vi "Init Rectangle.vi"(7 "Color (RGB black)":refnum<class "Color.lvclass">=refnum, 8 "error in (no error)":errorcluster, 9 "end point":cluster{"x":i16, "y":i16}, 10 "start point":cluster{"x":i16, "y":i16}, 11 "Rectangle in":refnum<class "Rectangle.lvclass">) -> (0 "error out":errorcluster, 3 "Rectangle out":refnum<class "Rectangle.lvclass">)   [LabVIEW 2020, in "Rectangle.lvclass"]
doc: "Initialize a rectangle"
uses:
  Rectangle.lvclass
  Color/Color.lvclass
  RGB Color/RGB Color.lvclass
panel:
  # "expressionflow.com"
  # "Copyright (c) 2008 Tomi Maila. All rights reserved."
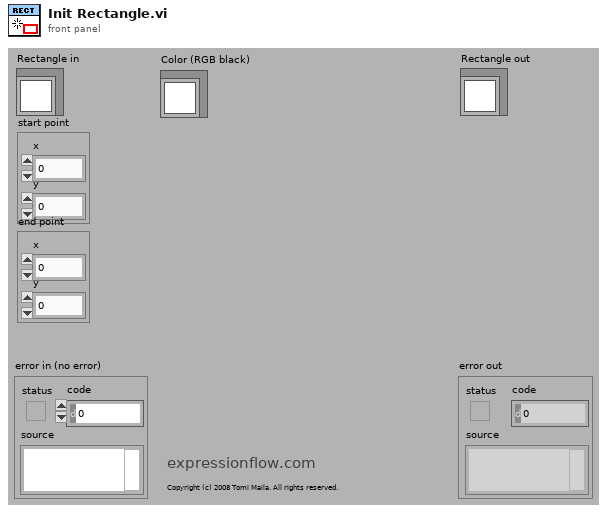
[diagram p1: front panel]
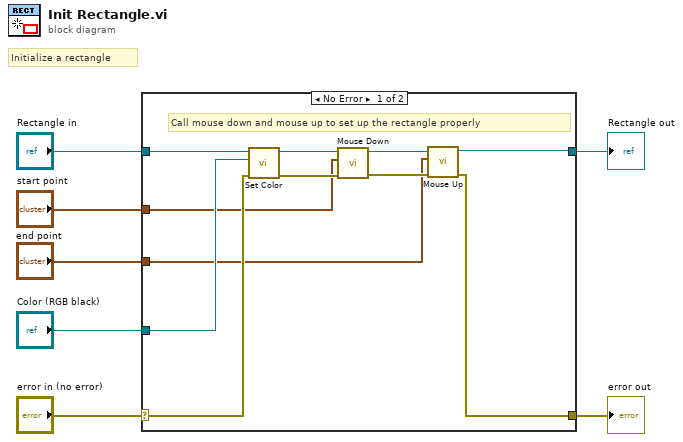
[diagram p0: block diagram]
diagram:
  # "Initialize a rectangle"
  n1 = case shown="No Error" "error in (no error)" {
    selector: "error in (no error)" -> [w17 w20]
    tunnel: [w8 w20] -> w6
    tunnel: [w13 w19] -> w4
    tunnel: "Rectangle in" -> [w18 w19]
    tunnel: "start point" -> [w10 _]
    tunnel: "end point" -> [w9 _]
    tunnel: "Color (RGB black)" -> [w16 _]
    frame No Error {
      # "Call mouse down and mouse up to set up the rectangle properly"
      n2 = call-dynamic "Set Color.vi"("error in (no error)"=w17, "Color (RGB black)"=w16, "Geometric Object.lvclass in"=w18) -> ("error out"=w11:errorcluster, "Geometric Object.lvclass out"=w15:refnum<class "Rectangle.lvclass">)  [unwired: 7 in]
      n3 = call-dynamic "Mouse Down.vi"("error in (no error)"=w11, "Point"=w10, "Geometric Object in"=w15) -> ("error out"=w12:errorcluster, "Geometric Object out"=w14:refnum<class "Rectangle.lvclass">)  [unwired: 7 in]
      n4 = call-dynamic "Mouse Up.vi"("error in (no error)"=w12, "Point"=w9, "Rectangle in"=w14) -> ("error out"=w8:errorcluster, "Rectangle out"=w13:refnum<class "Rectangle.lvclass">)  [unwired: 7 in]
    }
    frame Error {
    }
  }
  "error out" <- w6
  "Rectangle out" <- w4
